vi "wrap.PullBoolArray.vi"(0 "class.GLue in":refnum<class "class.GLue.lvclass">, 7 "Is2d":i32, 11 "error in (no error)":errorcluster, 13 "BoolArray in":bool[][](array[boolean])) -> (4 "class.GLue out":refnum<class "class.GLue.lvclass">, 8 "BoolArray out":bool[][](array[boolean]), 15 "error out":errorcluster)   [LabVIEW 2014, in "GLue.lvlib" / "class.GLue.lvclass"]
uses:
  class.GLue.lvclass
  class.GLue.lvclass/class.GLue.ctl
  Resources/GLue.dll
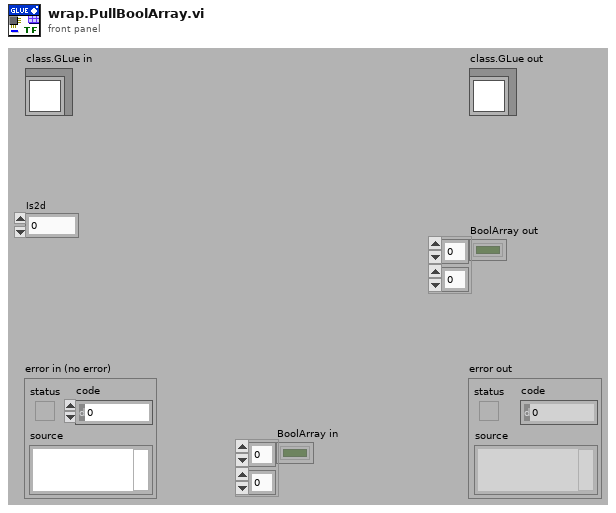
[diagram p1: front panel]
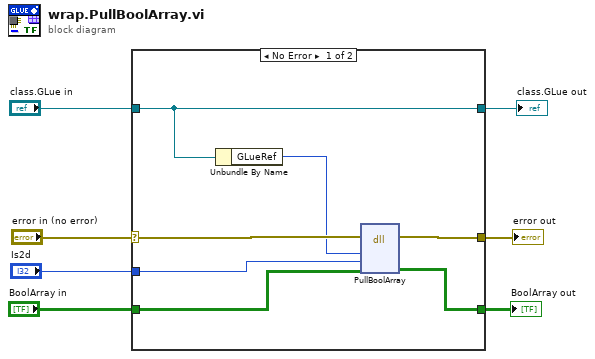
[diagram p0: block diagram]
diagram:
  n1 = case shown="No Error" "error in (no error)" {
    selector: "error in (no error)" -> [w13 w17]
    tunnel: [w12 w17] -> w6
    tunnel: [w14 w16] -> w4
    tunnel: "class.GLue in" -> [w14 w16]
    tunnel: "BoolArray in" -> [w10 w15]
    tunnel: [w9 w15] -> w2
    tunnel: "Is2d" -> [w8 _]
    frame No Error {
      n2 = Unbundle By Name(w14) -> ("GLueRef"=w11:i64)
      n3 = dll-call lib="C:/Users/Antonie/Documents/work/glue/trunk/Resources/GLue.dll" fn="PullBoolArray"(error in=w13, "MLua"=w11, "is2d"=w8, "BoolArray"=w10) -> (error out=w12:errorcluster, "BoolArray"=w9:bool[][])  [unwired: 5 in, 1 out]
    }
    frame Error {
    }
  }
  "error out" <- w6
  "class.GLue out" <- w4
  "BoolArray out" <- w2
